vi "Liquid Valve Control.vi"(0 "Session Handle in":T1, 5 "On?":bool=TRUE, 7 "Valve":i32, 11 "error in (no error)":errorcluster) -> (4 "Session Handle out":T1, 6 "Failure Reason":string, 8 "Success?":bool, 15 "error out":errorcluster)   [LabVIEW 2015, in "Oil.lvclass"]
uses:
  Oil.lvclass
  Typedefs/Session Handle.ctl
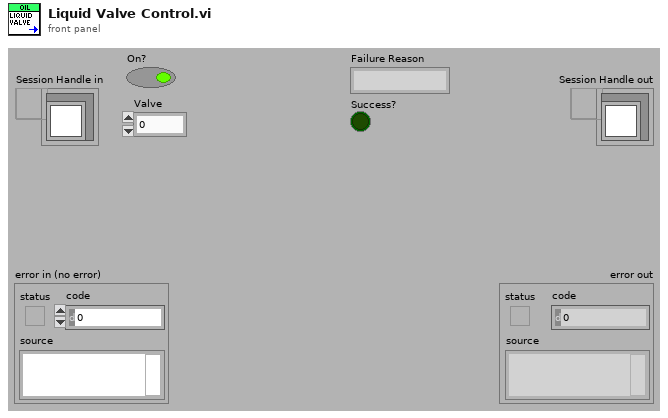
[diagram p1: front panel]
types:
  T1 = typedef "Oil.lvclass/Session Handle.ctl" = refnum<data-value>
  T2 = typedef "XNET Frame CAN.ctl" = cluster{"timestamp":timestamp, "payload":u8[], "identifier":u32, "type":T3, "extended?":bool, "echo?":bool}
  T3 = typedef "XNET Frame Type CAN.ctl" = u8
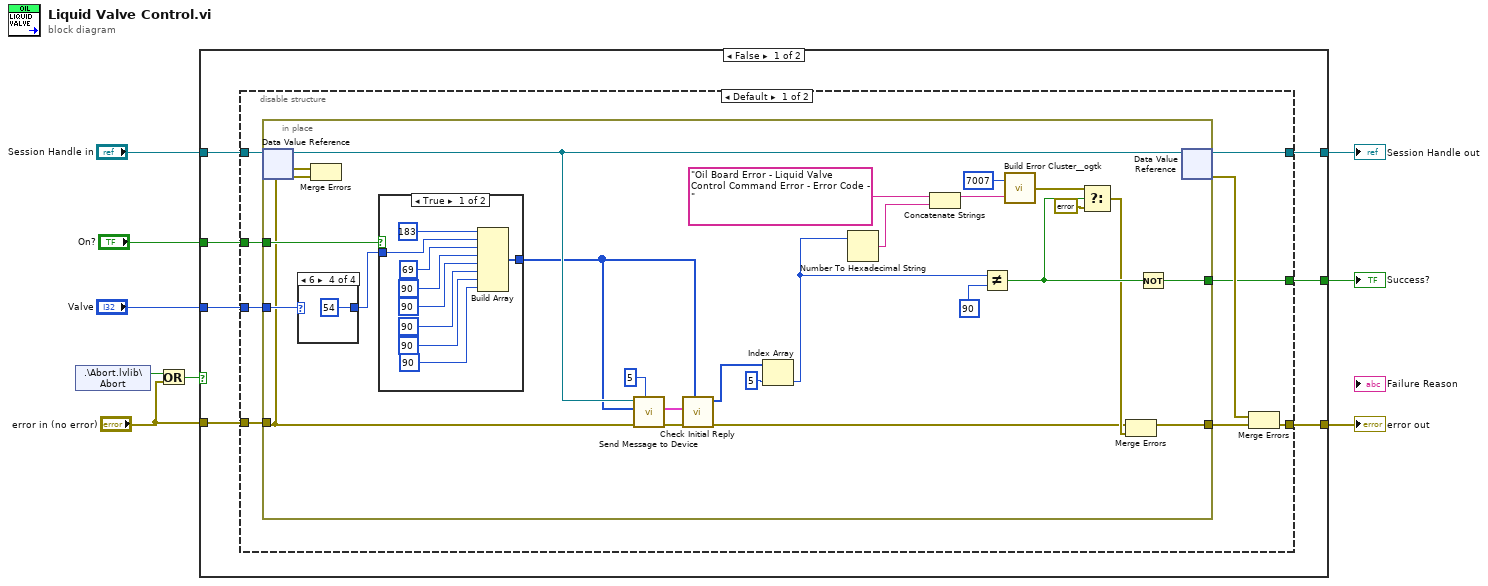
[diagram p0: block diagram]
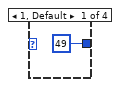
[diagram p2: hidden frame]
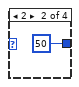
[diagram p3: hidden frame]
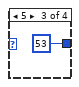
[diagram p4: hidden frame]
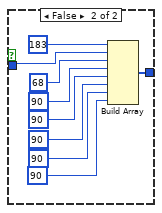
[diagram p5: hidden frame]
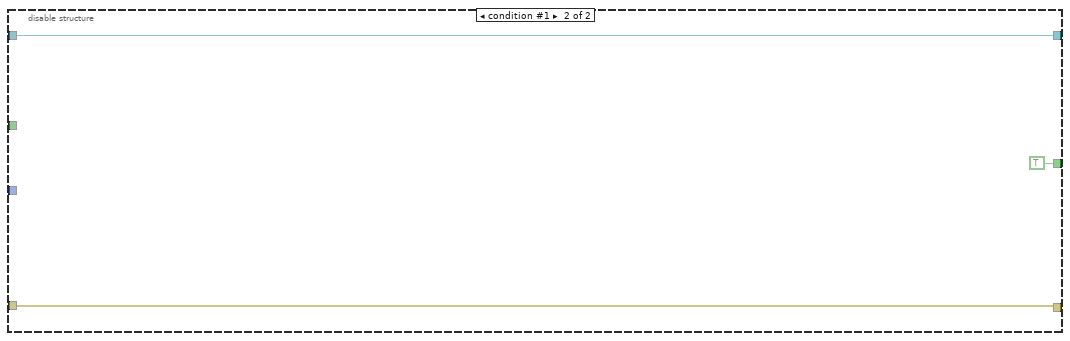
[diagram p6: hidden frame]
diagram:
  n1 = shared-variable ".\\Abort.lvlib\\Abort"() -> (w3:bool)  [unwired: 1 in, 1 out]
  n2 = Or(x=w3, y="error in (no error)") -> (x .or. y?=w2:bool)
  n3 = case shown="False" w2 {
    tunnel: "Session Handle in" -> [w16 w77]
    tunnel: [w15 w77] -> w8
    tunnel: [w14 w76] -> w7
    tunnel: "On?" -> [w13 _]
    tunnel: "Valve" -> [w12 _]
    tunnel: [w11 _] -> w4
    tunnel: "error in (no error)" -> [w10 w76]
    frame False {
      n4 = disable-structure shown="Default" {
        disable-tunnel: w16 -> [w25 w75]
        disable-tunnel: [w24 w75] -> w15
        disable-tunnel: [w22 w74] -> w14
        disable-tunnel: w13 -> [w21 _]
        disable-tunnel: w12 -> [w20 _]
        disable-tunnel: [w19 TRUE] -> w11
        disable-tunnel: w10 -> [w18 w74]
        frame condition #0 (active) {
          n5 = in-place {
            in-place-border: w21 -> [w45]
            in-place-border: w20 -> [w42]
            in-place-border: [w31] -> w19
            in-place-border: w18 -> [w29]
            in-place-border: [w28] -> w17
            n6 = in-place-dvr #1(w25) -> (w47:refnum<class "Oil.lvclass">, w50:errorcluster)
            n7 = case shown="6" w42 {
              tunnel: [u8 49 ("new element/subarray") u8 50 ("new element/subarray") u8 53 ("new element/subarray") u8 54 ("new element/subarray")] -> w41
              frame 1, Default {
              }
              frame 2 {
              }
              frame 5 {
              }
              frame 6 {
              }
            }
            n8 = Merge Errors(w29, w50) -> ()  [unwired: 1 out]
            n9 = case shown="True" w45 {
              tunnel: [w56 w65] -> w44
              tunnel: w41 -> [w55 w64]
              frame True {
                n10 = Build Array(u8 183 ("new element/subarray"), w55, u8 69 ("new element/subarray"), u8 90 ("new element/subarray"), u8 90 ("new element/subarray"), u8 90 ("new element/subarray"), u8 90 ("new element/subarray"), u8 90 ("new element/subarray")) -> (w56:u8[])
              }
              frame False {
                n11 = Build Array(u8 183 ("new element/subarray"), w64, u8 68 ("new element/subarray"), u8 90 ("new element/subarray"), u8 90 ("new element/subarray"), u8 90 ("new element/subarray"), u8 90 ("new element/subarray"), u8 90 ("new element/subarray")) -> (w65:u8[])
              }
            }
            n12 = call "Send Message to Device.vi"("Number of Retries"=5, "error in (no error)"=w29, "payload"=w44, "CAN Comm In"=w47) -> ("error out"=w27:errorcluster, "Reply"=w48:T2[])  [unwired: 5 in, 1 out]
            n13 = call "Check Initial Reply.vi"("Write Message"=w44, "error in (no error)"=w27, "Reply"=w48) -> ("error out"=w26:errorcluster, "Data Packet 2"=w46:u8[])  [unwired: 5 in, 2 out]
            n14 = Index Array(array=w46, index=5) -> (element=w32:u8)
            n15 = Number To Hexadecimal String(2:w32) -> (0:w34:string)  [unwired: 1 in]
            n16 = Concatenate Strings("Oil Board Error - Liquid Valve Control Command Error - Error Code - " ("string"), w34) -> (w39:string)
            n17 = Not Equal?(x=w32, y=u8 90 ("new element/subarray")) -> (x != y?=w35:bool)
            n18 = call <userlib>:"Build Error Cluster__ogtk.vi"("String to Prepend to source (\"\")"=w39, "code"=7007) -> ("error out"=w37:errorcluster)
            n19 = Select(t=w37, s=w35, f=errorcluster {"status"=FALSE, "code"=0, "source"=""}) -> (s? t:f=w30:errorcluster)
            n20 = Merge Errors(w26, w30) -> (w28:errorcluster)
            n21 = Not(x=w35) -> (.not. x?=w31:bool)
            n22 = in-place-dvr #1(w47) -> (w24:T1, w23:errorcluster)
          }
          n23 = Merge Errors(w23, w17) -> (w22:errorcluster)
        }
        frame condition #1 {
        }
      }
    }
    frame True {
    }
  }
  "Session Handle out" <- w8
  "error out" <- w7
  "Success?" <- w4
